vi "读取参数.vi"(8 "error in (no error)":errorcluster caption="错误输入（无错误）", 11 "设置文件路径":path) -> (0 "error out":errorcluster caption="错误输出", 3 "设置":T1)   [LabVIEW 2018]
uses:
  <vilib>/Utility/config.llb/Read Key (U32).vi
  <vilib>/Utility/config.llb/Read Key (String).vi
  <vilib>/Utility/config.llb/Read Key (Double).vi
  <vilib>/Utility/config.llb/Read Key (I32).vi
  <vilib>/Utility/config.llb/NI_LVConfig.lvlib
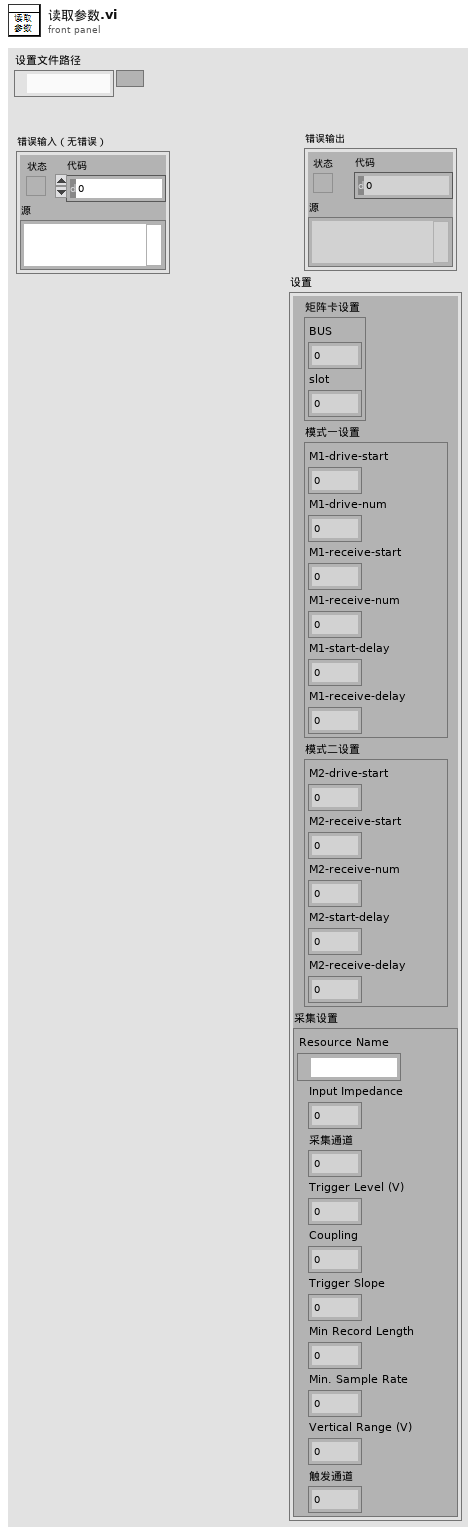
[diagram p1: front panel]
types:
  T1 = cluster{"矩阵卡设置":cluster{"BUS":u32, "slot":u32}, "模式一设置":cluster{"M1-drive-start":u32, "M1-drive-num":u32, "M1-receive-start":u32, "M1-receive-num":u32, "M1-start-delay":u32, "M1-receive-delay":u32}, "模式二设置":cluster{"M2-drive-start":u32, "M2-receive-start":u32, "M2-receive-num":u32, "M2-start-delay":u32, "M2-receive-delay":u32}, "采集设置":cluster{"Resource Name":refnum<k15>, "Input Impedance":u32, "采集通道":i32, "Trigger Level (V)":dbl, "Coupling":u16, "Trigger Slope":i32, "Min Record Length":i32, "Min. Sample Rate":dbl, "Vertical Range (V)":dbl, "触发通道":i32}}
  T2 = cluster{"Resource Name":refnum<k15>, "Input Impedance":u32, "采集通道":i32, "Trigger Level (V)":dbl, "Coupling":u16, "Trigger Slope":i32, "Min Record Length":i32, "Min. Sample Rate":dbl, "Vertical Range (V)":dbl, "触发通道":i32}
  T3 = cluster{"M1-drive-start":u32, "M1-drive-num":u32, "M1-receive-start":u32, "M1-receive-num":u32, "M1-start-delay":u32, "M1-receive-delay":u32}
  T4 = cluster{"M2-drive-start":u32, "M2-receive-start":u32, "M2-receive-num":u32, "M2-start-delay":u32, "M2-receive-delay":u32}
  T5 = typedef "NI_LVConfig.lvlib/Config Data RefNum.ctl" = refnum<k1>
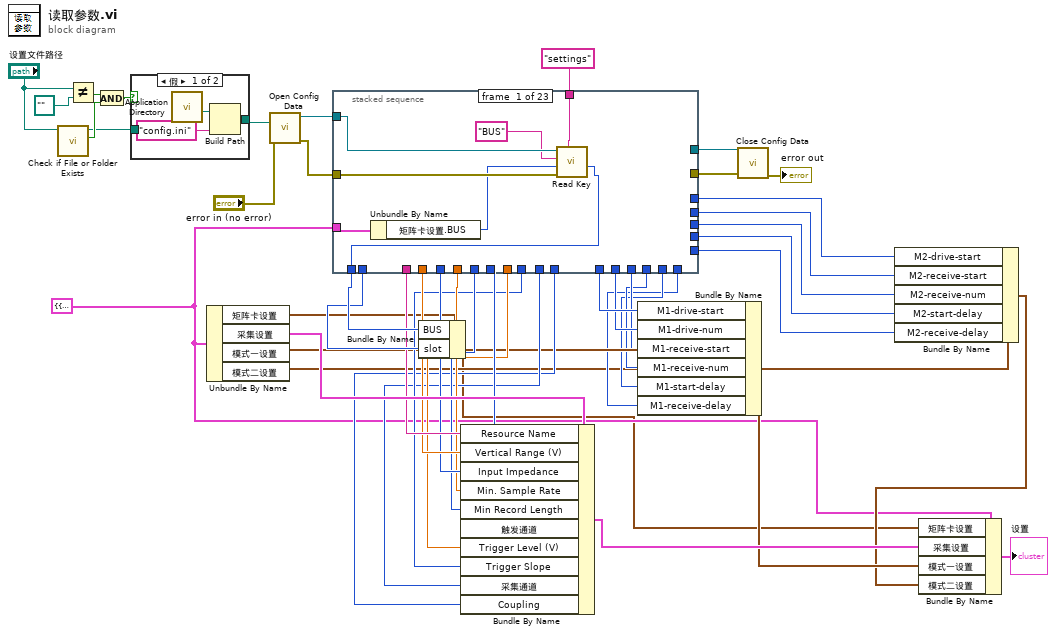
[diagram p0: block diagram]
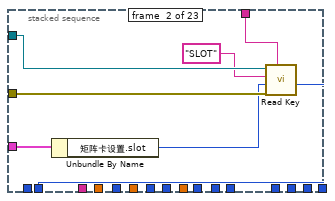
[diagram p3: hidden frame]
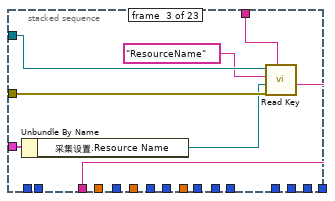
[diagram p4: hidden frame]
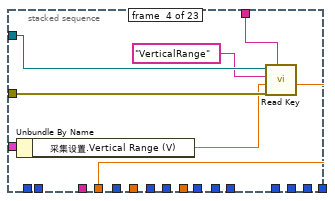
[diagram p5: hidden frame]
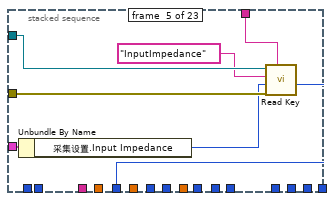
[diagram p6: hidden frame]
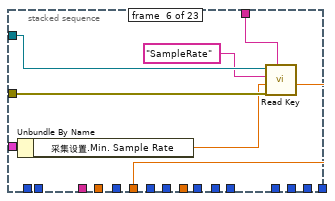
[diagram p7: hidden frame]
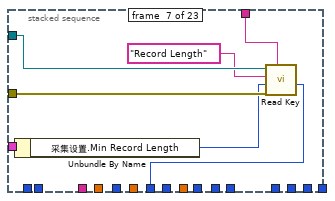
[diagram p8: hidden frame]
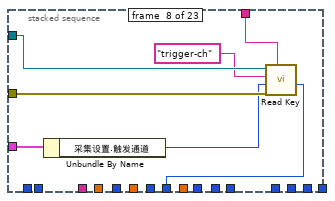
[diagram p9: hidden frame]
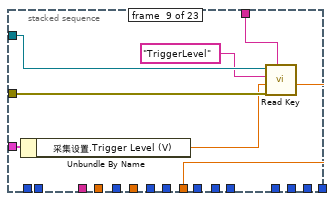
[diagram p10: hidden frame]
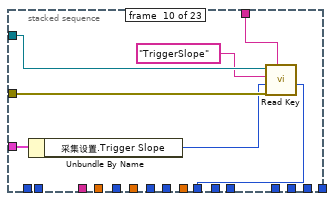
[diagram p11: hidden frame]
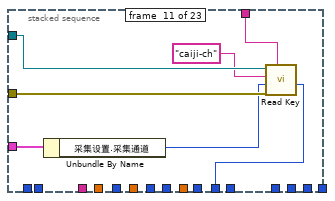
[diagram p12: hidden frame]
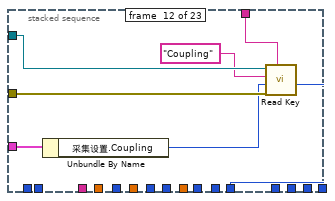
[diagram p13: hidden frame]
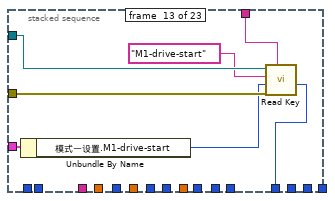
[diagram p14: hidden frame]
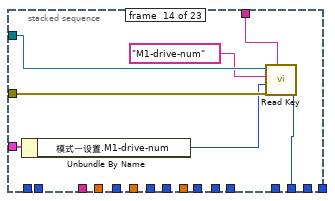
[diagram p15: hidden frame]
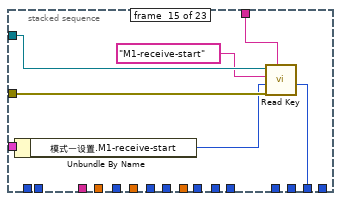
[diagram p16: hidden frame]
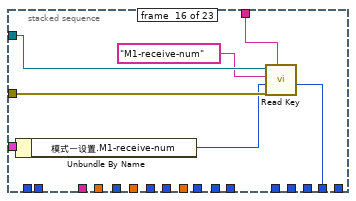
[diagram p17: hidden frame]
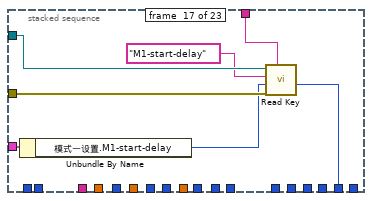
[diagram p18: hidden frame]
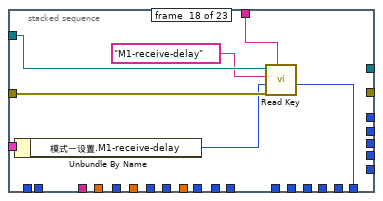
[diagram p19: hidden frame]
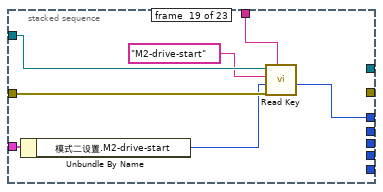
[diagram p20: hidden frame]
diagram:
  w3 = T1 {"矩阵卡设置"={"BUS"=0, "slot"=0}, "模式一设置"={"M1-drive-start"=0, "M1-drive-num"=0, "M1-receive-start"=0, "M1-receive-num"=0, "M1-start-delay"=0, "M1-receive-delay"=0}, "模式二设置"={"M2-drive-start"=0, "M2-receive-start"=0, "M2-receive-num"=0, "M2-start-delay"=0, "M2-receive-delay"=0}, "采集设置"={"Resource Name"="", "Input Impedance"=0, "采集通道"=0, "Trigger Level (V)"=0.0, "Coupling"=0, "Trigger Slope"=0, "Min Record Length"=0, "Min. Sample Rate"=0.0, "Vertical Range (V)"=0.0, "触发通道"=0}} ("设置")
  n1 = call <vilib>:"Check if File or Folder Exists.vi"("path"="设置文件路径") -> ("file or folder exists?"=w6:bool, "dup path"=w4:path)  [unwired: 8 in, 1 out]
  n2 = Not Equal?(x="设置文件路径", y=path "" ("添加的路径")) -> (x != y?=w7:bool)
  n3 = And(x=w7, y=w6) -> (x .and. y?=w5:bool)
  n4 = case shown="假" w5 {
    tunnel: [w48 w51] -> w10
    tunnel: w4 -> [_ w51]
    frame False {
      n5 = call <vilib>:"Application Directory.vi"() -> ("Application Directory"=w50:path)
      n6 = Build Path(base path=w50, name or relative path="config.ini" ("名称或相对路径")) -> (appended path=w48:path)
    }
    frame True {
    }
  }
  n7 = Unbundle By Name(w3) -> ("矩阵卡设置"=w14:cluster{"BUS":u32, "slot":u32}, "采集设置"=w38:T2, "模式一设置"=w27:T3, "模式二设置"=w20:T4)
  n8 = call <vilib>:"Open Config Data.vi"("error in (no error)"="error in (no error)", "configuration file path"=w10) -> ("error out"=w46:errorcluster, "refnum"=w47:T5)  [unwired: 7 in, 1 out]
  n9 = stacked-sequence {
    tunnel: w47 -> [w56 w64 w71 w78 w85 w92 w99 w106 w113 w120 w127 w134 w141 w148 w155 w162 w169 w176 w183 w190 w197 w204 w213]
    tunnel: w46 -> [w57 w63 w70 w77 w84 w91 w98 w105 w112 w119 w126 w133 w140 w147 w154 w161 w168 w175 w182 w189 w196 w203 w212]
    tunnel: "settings" ("section") -> [w58 w65 w72 w79 w86 w93 w100 w107 w114 w121 w128 w135 w142 w149 w156 w163 w170 w177 w184 w191 w198 w205 w214]
    tunnel: w3 -> [w55 w62 w69 w76 w83 w90 w97 w104 w111 w118 w125 w132 w139 w146 w153 w160 w167 w174 w181 w188 w195 w202 w211]
    tunnel: [_ _ _ _ _ _ _ _ _ _ _ _ _ _ _ _ _ _ _ _ _ _ w208] -> w44
    tunnel: [_ _ _ _ _ _ _ _ _ _ _ _ _ _ _ _ _ _ _ _ _ _ w207] -> w43
    tunnel: [w52 _ _ _ _ _ _ _ _ _ _ _ _ _ _ _ _ _ _ _ _ _ _] -> w40
    tunnel: [_ w59 _ _ _ _ _ _ _ _ _ _ _ _ _ _ _ _ _ _ _ _ _] -> w39
    tunnel: [_ _ w66 _ _ _ _ _ _ _ _ _ _ _ _ _ _ _ _ _ _ _ _] -> w37
    tunnel: [_ _ _ w73 _ _ _ _ _ _ _ _ _ _ _ _ _ _ _ _ _ _ _] -> w36
    tunnel: [_ _ _ _ w80 _ _ _ _ _ _ _ _ _ _ _ _ _ _ _ _ _ _] -> w35
    tunnel: [_ _ _ _ _ w87 _ _ _ _ _ _ _ _ _ _ _ _ _ _ _ _ _] -> w34
    tunnel: [_ _ _ _ _ _ w94 _ _ _ _ _ _ _ _ _ _ _ _ _ _ _ _] -> w33
    tunnel: [_ _ _ _ _ _ _ w101 _ _ _ _ _ _ _ _ _ _ _ _ _ _ _] -> w32
    tunnel: [_ _ _ _ _ _ _ _ w108 _ _ _ _ _ _ _ _ _ _ _ _ _ _] -> w31
    tunnel: [_ _ _ _ _ _ _ _ _ w115 _ _ _ _ _ _ _ _ _ _ _ _ _] -> w30
    tunnel: [_ _ _ _ _ _ _ _ _ _ w122 _ _ _ _ _ _ _ _ _ _ _ _] -> w29
    tunnel: [_ _ _ _ _ _ _ _ _ _ _ w129 _ _ _ _ _ _ _ _ _ _ _] -> w28
    tunnel: [_ _ _ _ _ _ _ _ _ _ _ _ w136 _ _ _ _ _ _ _ _ _ _] -> w26
    tunnel: [_ _ _ _ _ _ _ _ _ _ _ _ _ w143 _ _ _ _ _ _ _ _ _] -> w25
    tunnel: [_ _ _ _ _ _ _ _ _ _ _ _ _ _ w150 _ _ _ _ _ _ _ _] -> w24
    tunnel: [_ _ _ _ _ _ _ _ _ _ _ _ _ _ _ w157 _ _ _ _ _ _ _] -> w23
    tunnel: [_ _ _ _ _ _ _ _ _ _ _ _ _ _ _ _ w164 _ _ _ _ _ _] -> w22
    tunnel: [_ _ _ _ _ _ _ _ _ _ _ _ _ _ _ _ _ w171 _ _ _ _ _] -> w21
    tunnel: [_ _ _ _ _ _ _ _ _ _ _ _ _ _ _ _ _ _ w178 _ _ _ _] -> w19
    tunnel: [_ _ _ _ _ _ _ _ _ _ _ _ _ _ _ _ _ _ _ w185 _ _ _] -> w18
    tunnel: [_ _ _ _ _ _ _ _ _ _ _ _ _ _ _ _ _ _ _ _ w192 _ _] -> w17
    tunnel: [_ _ _ _ _ _ _ _ _ _ _ _ _ _ _ _ _ _ _ _ _ w199 _] -> w16
    tunnel: [_ _ _ _ _ _ _ _ _ _ _ _ _ _ _ _ _ _ _ _ _ _ w206] -> w15
    frame #0 {
      n10 = Unbundle By Name(w55) -> ("矩阵卡设置.BUS"=w53:u32)
      n11 = call-poly <vilib>:"Read Key.vi"("section"=w58, "error in (no error)"=w57, "default value"=w53, "key"="BUS", "refnum"=w56) -> ("value"=w52:u32)  [unwired: 3 in, 3 out]
    }
    frame #1 {
      n12 = Unbundle By Name(w62) -> ("矩阵卡设置.slot"=w60:u32)
      n13 = call-poly <vilib>:"Read Key.vi"("section"=w65, "error in (no error)"=w63, "default value"=w60, "key"="SLOT", "refnum"=w64) -> ("value"=w59:u32)  [unwired: 3 in, 3 out]
    }
    frame #2 {
      n14 = Unbundle By Name(w69) -> ("采集设置.Resource Name"=w67:refnum<k15>)
      n15 = call-poly <vilib>:"Read Key.vi"("section"=w72, "error in (no error)"=w70, "default value"=w67, "key"="ResourceName", "refnum"=w71) -> ("value"=w66:string)  [unwired: 3 in, 3 out]
    }
    frame #3 {
      n16 = Unbundle By Name(w76) -> ("采集设置.Vertical Range (V)"=w74:dbl)
      n17 = call-poly <vilib>:"Read Key.vi"("section"=w79, "error in (no error)"=w77, "default value"=w74, "key"="VerticalRange", "refnum"=w78) -> ("value"=w73:dbl)  [unwired: 3 in, 3 out]
    }
    frame #4 {
      n18 = Unbundle By Name(w83) -> ("采集设置.Input Impedance"=w81:u32)
      n19 = call-poly <vilib>:"Read Key.vi"("section"=w86, "error in (no error)"=w84, "default value"=w81, "key"="InputImpedance", "refnum"=w85) -> ("value"=w80:u32)  [unwired: 3 in, 3 out]
    }
    frame #5 {
      n20 = Unbundle By Name(w90) -> ("采集设置.Min. Sample Rate"=w88:dbl)
      n21 = call-poly <vilib>:"Read Key.vi"("section"=w93, "error in (no error)"=w91, "default value"=w88, "key"="SampleRate", "refnum"=w92) -> ("value"=w87:dbl)  [unwired: 3 in, 3 out]
    }
    frame #6 {
      n22 = Unbundle By Name(w97) -> ("采集设置.Min Record Length"=w95:i32)
      n23 = call-poly <vilib>:"Read Key.vi"("section"=w100, "error in (no error)"=w98, "default value"=w95, "key"="Record Length", "refnum"=w99) -> ("value"=w94:i32)  [unwired: 3 in, 3 out]
    }
    frame #7 {
      n24 = Unbundle By Name(w104) -> ("采集设置.触发通道"=w102:i32)
      n25 = call-poly <vilib>:"Read Key.vi"("section"=w107, "error in (no error)"=w105, "default value"=w102, "key"="trigger-ch", "refnum"=w106) -> ("value"=w101:i32)  [unwired: 3 in, 3 out]
    }
    frame #8 {
      n26 = Unbundle By Name(w111) -> ("采集设置.Trigger Level (V)"=w109:dbl)
      n27 = call-poly <vilib>:"Read Key.vi"("section"=w114, "error in (no error)"=w112, "default value"=w109, "key"="TriggerLevel", "refnum"=w113) -> ("value"=w108:dbl)  [unwired: 3 in, 3 out]
    }
    frame #9 {
      n28 = Unbundle By Name(w118) -> ("采集设置.Trigger Slope"=w116:i32)
      n29 = call-poly <vilib>:"Read Key.vi"("section"=w121, "error in (no error)"=w119, "default value"=w116, "key"="TriggerSlope", "refnum"=w120) -> ("value"=w115:i32)  [unwired: 3 in, 3 out]
    }
    frame #10 {
      n30 = Unbundle By Name(w125) -> ("采集设置.采集通道"=w123:i32)
      n31 = call-poly <vilib>:"Read Key.vi"("section"=w128, "error in (no error)"=w126, "default value"=w123, "key"="caiji-ch", "refnum"=w127) -> ("value"=w122:i32)  [unwired: 3 in, 3 out]
    }
    frame #11 {
      n32 = Unbundle By Name(w132) -> ("采集设置.Coupling"=w130:u16)
      n33 = call-poly <vilib>:"Read Key.vi"("section"=w135, "error in (no error)"=w133, "default value"=w130, "key"="Coupling", "refnum"=w134) -> ("value"=w129:u32)  [unwired: 3 in, 3 out]
    }
    frame #12 {
      n34 = Unbundle By Name(w139) -> ("模式一设置.M1-drive-start"=w137:u32)
      n35 = call-poly <vilib>:"Read Key.vi"("section"=w142, "error in (no error)"=w140, "default value"=w137, "key"="M1-drive-start", "refnum"=w141) -> ("value"=w136:u32)  [unwired: 3 in, 3 out]
    }
    frame #13 {
      n36 = Unbundle By Name(w146) -> ("模式一设置.M1-drive-num"=w144:u32)
      n37 = call-poly <vilib>:"Read Key.vi"("section"=w149, "error in (no error)"=w147, "default value"=w144, "key"="M1-drive-num", "refnum"=w148) -> ("value"=w143:u32)  [unwired: 3 in, 3 out]
    }
    frame #14 {
      n38 = Unbundle By Name(w153) -> ("模式一设置.M1-receive-start"=w151:u32)
      n39 = call-poly <vilib>:"Read Key.vi"("section"=w156, "error in (no error)"=w154, "default value"=w151, "key"="M1-receive-start", "refnum"=w155) -> ("value"=w150:u32)  [unwired: 3 in, 3 out]
    }
    frame #15 {
      n40 = Unbundle By Name(w160) -> ("模式一设置.M1-receive-num"=w158:u32)
      n41 = call-poly <vilib>:"Read Key.vi"("section"=w163, "error in (no error)"=w161, "default value"=w158, "key"="M1-receive-num", "refnum"=w162) -> ("value"=w157:u32)  [unwired: 3 in, 3 out]
    }
    frame #16 {
      n42 = Unbundle By Name(w167) -> ("模式一设置.M1-start-delay"=w165:u32)
      n43 = call-poly <vilib>:"Read Key.vi"("section"=w170, "error in (no error)"=w168, "default value"=w165, "key"="M1-start-delay", "refnum"=w169) -> ("value"=w164:u32)  [unwired: 3 in, 3 out]
    }
    frame #17 {
      n44 = Unbundle By Name(w174) -> ("模式一设置.M1-receive-delay"=w172:u32)
      n45 = call-poly <vilib>:"Read Key.vi"("section"=w177, "error in (no error)"=w175, "default value"=w172, "key"="M1-receive-delay", "refnum"=w176) -> ("value"=w171:u32)  [unwired: 3 in, 3 out]
    }
    frame #18 {
      n46 = Unbundle By Name(w181) -> ("模式二设置.M2-drive-start"=w179:u32)
      n47 = call-poly <vilib>:"Read Key.vi"("section"=w184, "error in (no error)"=w182, "default value"=w179, "key"="M2-drive-start", "refnum"=w183) -> ("value"=w178:u32)  [unwired: 3 in, 3 out]
    }
    frame #19 {
      n48 = Unbundle By Name(w188) -> ("模式二设置.M2-receive-start"=w186:u32)
      n49 = call-poly <vilib>:"Read Key.vi"("section"=w191, "error in (no error)"=w189, "default value"=w186, "key"="M2-receive-start", "refnum"=w190) -> ("value"=w185:u32)  [unwired: 3 in, 3 out]
    }
    frame #20 {
      n50 = Unbundle By Name(w195) -> ("模式二设置.M2-receive-num"=w193:u32)
      n51 = call-poly <vilib>:"Read Key.vi"("section"=w198, "error in (no error)"=w196, "default value"=w193, "key"="M2-receive-num", "refnum"=w197) -> ("value"=w192:u32)  [unwired: 3 in, 3 out]
    }
    frame #21 {
      n52 = Unbundle By Name(w202) -> ("模式二设置.M2-start-delay"=w200:u32)
      n53 = call-poly <vilib>:"Read Key.vi"("section"=w205, "error in (no error)"=w203, "default value"=w200, "key"="M2-start-delay", "refnum"=w204) -> ("value"=w199:u32)  [unwired: 3 in, 3 out]
    }
    frame #22 {
      n54 = Unbundle By Name(w211) -> ("模式二设置.M2-receive-delay"=w209:u32)
      n55 = call-poly <vilib>:"Read Key.vi"("section"=w214, "error in (no error)"=w212, "default value"=w209, "key"="M2-receive-delay", "refnum"=w213) -> ("error out"=w207:errorcluster, "value"=w206:u32, "refnum out"=w208:T5)  [unwired: 3 in, 1 out]
    }
  }
  n56 = Bundle By Name(cluster=w14, "BUS"=w40, "slot"=w39) -> (w1:cluster{"BUS":u32, "slot":u32})
  n57 = Bundle By Name(cluster=w38, "Resource Name"=w37, "Vertical Range (V)"=w36, "Input Impedance"=w35, "Min. Sample Rate"=w34, "Min Record Length"=w33, "触发通道"=w32, "Trigger Level (V)"=w31, "Trigger Slope"=w30, "采集通道"=w29, "Coupling"=w28) -> (w13:T2)
  n58 = Bundle By Name(cluster=w27, "M1-drive-start"=w26, "M1-drive-num"=w25, "M1-receive-start"=w24, "M1-receive-num"=w23, "M1-start-delay"=w22, "M1-receive-delay"=w21) -> (w12:T3)
  n59 = call <vilib>:"Close Config Data.vi"("error in (no error)"=w43, "refnum"=w44) -> ("error out"=→"error out":errorcluster)  [unwired: 8 in, 1 out]
  n60 = Bundle By Name(cluster=w20, "M2-drive-start"=w19, "M2-receive-start"=w18, "M2-receive-num"=w17, "M2-start-delay"=w16, "M2-receive-delay"=w15) -> (w11:T4)
  n61 = Bundle By Name(cluster=w3, "矩阵卡设置"=w1, "采集设置"=w13, "模式一设置"=w12, "模式二设置"=w11) -> (→"设置":T1)
